vi "PR_CAN_Labview_Demo.vi"() -> ()   [LabVIEW 2017]
uses:
  Fuse25A_Labview/Power-Rider-GUI/CANalystII/PCAN_Driver/ControlCAN.llb/CAN Channel.ctl
  D:/Projects/GUI/Power Rider Wrapper/PowerRiderDLLWrapper.dll
  PowerRiderDLLWrapper.dll
  Fuse25A_Labview/Power-Rider-GUI/CANalystII/PCAN_Driver/ControlCAN.lvlib
panel:
  in  "Channel #":T1 caption="Channel" items=["Channel 1", "Channel 2"]
  in  "Baud":u32(ring)=250000 items=["1M"=1000000, "800K"=800000, "500K"=500000, "250K"=250000, "125K"=125000, "100K"=100000, "83.3K"=83300, "50000"=50000, "20K"=20000, "10K"=10000, "5K"=5000]
  in  "String":string
  out "CommIcon":bool
  in  "Dst add":u16=16
  in  "address":u16=85
  in  "TripType Enum":T2(ring)
  in  "Status Enum":enum16{"OFF", "ON", "ERROR", "FOREVER OFF"}(ring)
  # "Power Rider Demo"
  # "CANalytst-II interface"
  # "ver 1.0"
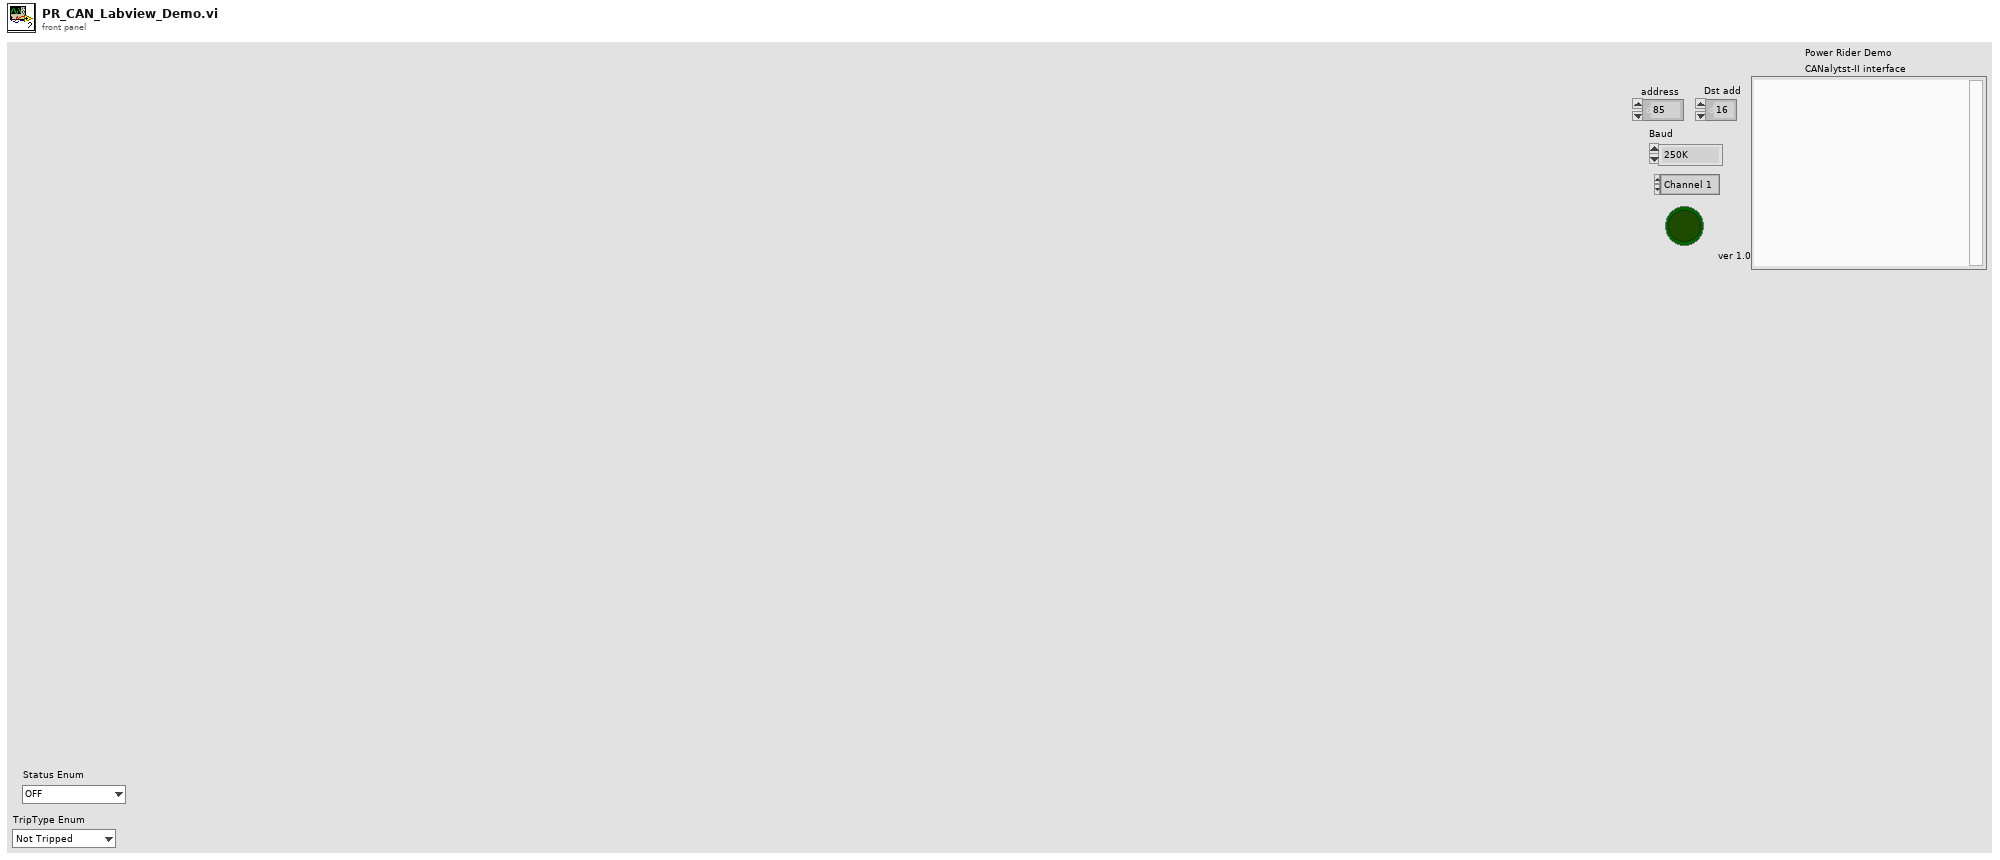
[diagram p1: front panel]
types:
  T1 = typedef "ControlCAN.lvlib/CAN Channel.ctl" = u32
  T2 = enum16{"Not Tripped", "SW Tripped", "Hard Short", "MAX SW Tripped"}
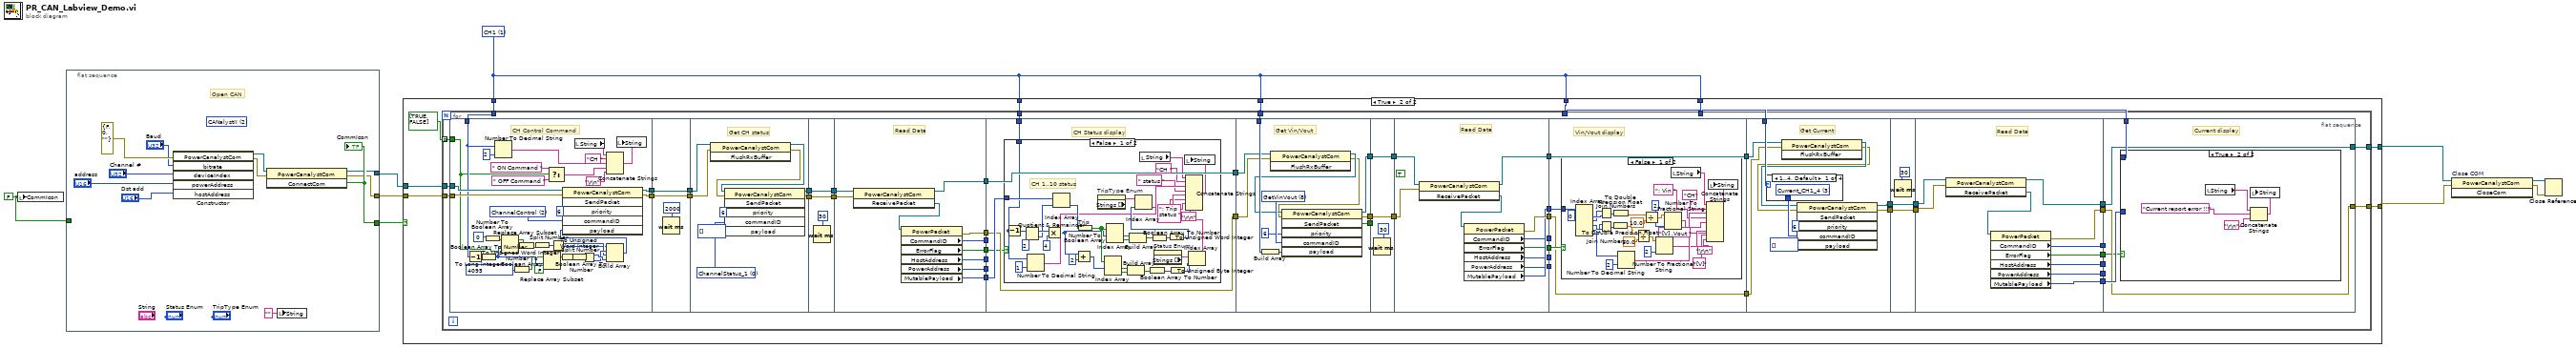
[diagram p0: block diagram]
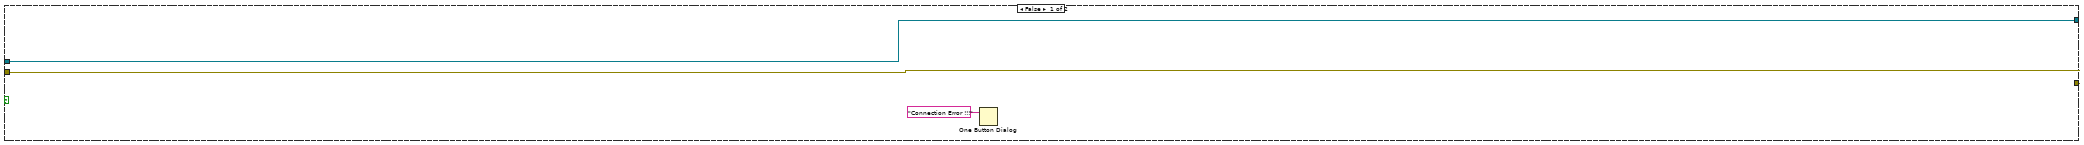
[diagram p2: hidden frame]
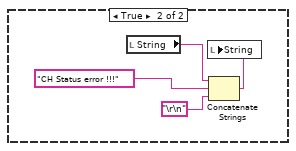
[diagram p3: hidden frame]
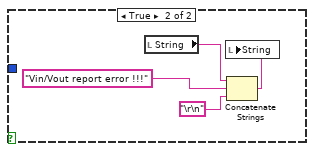
[diagram p4: hidden frame]
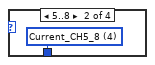
[diagram p5: hidden frame]
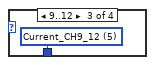
[diagram p6: hidden frame]
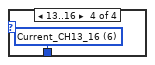
[diagram p7: hidden frame]
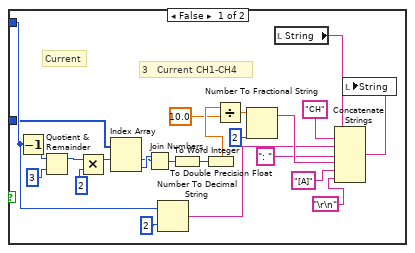
[diagram p8: hidden frame]
diagram:
  w1 = FALSE ("CommIcon")
  w6 = u8 1 items=["CH1"=1, "CH2"=2, "CH3"=3, "CH4"=4, "CH5"=5, "CH6"=6, "CH7"=7, "CH8"=8, "CH9"=9, "CH10"=10, "CH11"=11, "CH12"=12, "CH13"=13, "CH14"=14, "CH15"=15, "CH16"=16] ("Select CH #")
  n1 = local write "CommIcon"(w1) -> ()
  n2 = flat-sequence {
    tunnel: [w12] -> w9
    tunnel: [w11] -> w3
    tunnel: [w10] -> w2
    tunnel: w1 -> [_]
    frame #0 {
      (unwired) u16 2 items=["CANalystII"=2, "TCP Client"=3, "TCP Server"=4, "UDP Client"=5, "Serial COM"=6, "CAN Kvaser"=7] ("COMType 2")
      # "Open CAN"
      n3 = constructor class="PowerCanalystCom"(error in=errorcluster {"status"=FALSE, "code"=0, "source"=""} ("error out"), "bitrate"="Baud", "deviceIndex"="Channel #", "powerAddress"="address", "hostAddress"="Dst add") -> (reference out=w13:refnum<k24>, error out=w14:errorcluster)  [unwired: 2 in, 5 out]
      n4 = invoke class="PowerCanalystCom" method="ConnectCom"(reference=w13, error in=w14) -> (reference out=w10:refnum<k24>, error out=w11:errorcluster, "ConnectCom"=w12:bool)  [unwired: 1 in]
      "CommIcon" <- w12
      n5 = local write "String"("" ("String")) -> ()
    }
  }
  n6 = case shown="True" w9 {
    tunnel: w2 -> [w22 w28]
    tunnel: w3 -> [w23 w27]
    tunnel: w6 -> [_ w33]
    tunnel: w6 -> [_ w32]
    tunnel: w6 -> [_ w31]
    tunnel: w6 -> [_ w30]
    tunnel: w6 -> [_ w29]
    tunnel: [w22 w26] -> w5
    tunnel: [w23 w25] -> w4
    frame False {
      n7 = One Button Dialog(message="Connection Error !!!") -> ()  [unwired: 1 in, 1 out]
    }
    frame True {
      n8 = for {
        tunnel: w33 -> [w34]
        tunnel: w32 -> [w74]
        tunnel: w31 -> [w73]
        tunnel: w30 -> [w72]
        tunnel: w29 -> [w35]
        tunnel: w28 -> [w71]
        tunnel: w27 -> [w70]
        tunnel: [w69] -> w26
        tunnel: [w68] -> w25
        tunnel: bool[] [TRUE, FALSE] -> [w67] mode=indexing
        n9 = flat-sequence {
          tunnel: w70 -> [w99]
          tunnel: [w101] -> w85
          tunnel: [w100] -> w84
          tunnel: w35 -> [w94]
          tunnel: w71 -> [w98]
          tunnel: w67 -> [w90]
          tunnel: w85 -> [w123]
          tunnel: [w123] -> w83
          tunnel: w84 -> [w122]
          tunnel: [w122] -> w82
          tunnel: [w129] -> w66
          tunnel: [w128] -> w64
          tunnel: w83 -> [w127]
          tunnel: w82 -> [w126]
          tunnel: w66 -> [w135]
          tunnel: [w135] -> w65
          tunnel: w64 -> [w134]
          tunnel: [w134] -> w63
          tunnel: w65 -> [w142]
          tunnel: w63 -> [w143]
          tunnel: [w145] -> w81
          tunnel: [w144] -> w80
          tunnel: [w140] -> w79
          tunnel: [w139] -> w48
          tunnel: [w138] -> w47
          tunnel: [w137] -> w46
          tunnel: [w136] -> w45
          tunnel: w81 -> [w148]
          tunnel: w80 -> [w150]
          tunnel: w79 -> [w149]
          tunnel: [w149] -> w78
          tunnel: [w148] -> w77
          tunnel: w34 -> [w147]
          tunnel: w48 -> [w146]
          tunnel: w47 -> [_]
          tunnel: w46 -> [_]
          tunnel: w45 -> [_]
          tunnel: w78 -> [w192]
          tunnel: w77 -> [w190]
          tunnel: w74 -> [w194]
          tunnel: [w196] -> w62
          tunnel: [w195] -> w61
          tunnel: [w193] -> w44
          tunnel: w62 -> [w202]
          tunnel: [w202] -> w59
          tunnel: w61 -> [w201]
          tunnel: [w201] -> w57
          tunnel: w44 -> [_]
          tunnel: [w211] -> w60
          tunnel: w59 -> [w209]
          tunnel: [w208] -> w58
          tunnel: w57 -> [w210]
          tunnel: [w212] -> w56
          tunnel: [w206] -> w43
          tunnel: [w205] -> w42
          tunnel: [w204] -> w41
          tunnel: [w203] -> w40
          tunnel: w60 -> [w216]
          tunnel: [w215] -> w76
          tunnel: w58 -> [w215]
          tunnel: w56 -> [w213]
          tunnel: [w213] -> w75
          tunnel: w43 -> [_]
          tunnel: w42 -> [w214]
          tunnel: w41 -> [_]
          tunnel: w40 -> [_]
          tunnel: w73 -> [w257]
          tunnel: w76 -> [w252]
          tunnel: w75 -> [w251]
          tunnel: [w254] -> w55
          tunnel: [w253] -> w54
          tunnel: w55 -> [w265]
          tunnel: [w265] -> w53
          tunnel: w54 -> [w264]
          tunnel: [w264] -> w51
          tunnel: w53 -> [w273]
          tunnel: [w274] -> w52
          tunnel: w51 -> [w272]
          tunnel: [w270] -> w50
          tunnel: [w275] -> w49
          tunnel: [w269] -> w39
          tunnel: [w268] -> w38
          tunnel: [w267] -> w37
          tunnel: [w266] -> w36
          tunnel: w52 -> [w277]
          tunnel: w50 -> [w278]
          tunnel: w72 -> [w280]
          tunnel: w49 -> [w279]
          tunnel: [w278] -> w69
          tunnel: [w277] -> w68
          tunnel: w39 -> [w276]
          tunnel: w38 -> [_]
          tunnel: w37 -> [_]
          tunnel: w36 -> [_]
          frame #0 {
            w102 = u8 2 items=["ChannelStatus_1"=0, "ChannelControl"=2, "Current_CH1_4"=3, "Current_CH5_8"=4, "Current_CH9_12"=5, "Current_CH13_16"=6, "GetVinVout"=8, "Version_BoardType"=9, "SystemTemp"=10, "SystemParameter"=11, "ChannelParameter"=12, "GetTripEvent"=15, "LogFile"=18, "Configuration"=19, "ProductionData"=20, "BIT"=33, "DiscretePorts"=34, "SerialNumber"=36, "OffsetMeasurement"=37, "PartNumber"=39, "ChannelCombinedStatus_1_CH1_8"=40, "ChannelCombinedStatus_2_CH9_12"=41, "PlotData"=45, "PlotCommand"=46, "InternalData"=47, "KeepAlive"=234, "WakeUp"=250] ("commandID")
            # "CH Control Command"
            n10 = Decrement(x=w94) -> (x-1=w103:u8)
            n11 = To Long Integer(number=w103) -> (32bit integer=w109:i32)
            n12 = Number To Boolean Array(number=u16 0 ("element")) -> (Boolean array=w105:bool[])
            n13 = Number To Decimal String(number=w94, width (-)=i16 2) -> (decimal integer string=w91:string)
            n14 = Replace Array Subset(array=w105, new element=w90, index=w109) -> (w106:bool[])
            n15 = Number To Boolean Array(number=u16 4095 ("mask")) -> (Boolean array=w108:bool[])
            n16 = Boolean Array To Number(Boolean array=w106) -> (number=w107:u32)
            n17 = To Unsigned Word Integer(number=w107) -> (unsigned 16bit integer=w114:u16)
            n18 = Replace Array Subset(array=w108, new element=FALSE ("new element/subarray"), index=w109) -> (w104:bool[])
            n19 = Select(t=" ON Command " ("string"), s=w90, f=" OFF Command " ("string")) -> (s? t:f=w87:string)
            n20 = Split Number(x=w114) -> (hi(x)=w118:u8, lo(x)=w117:u8)
            n21 = Boolean Array To Number(Boolean array=w104) -> (number=w113:u32)
            n22 = To Unsigned Word Integer(number=w113) -> (unsigned 16bit integer=w116:u16)
            n23 = local read "String"() -> (w96:string)
            n24 = Split Number(x=w116) -> (hi(x)=w120:u8, lo(x)=w119:u8)
            n25 = Concatenate Strings(w96, "CH " ("string"), w91, w87, "\r\n") -> (w95:string)
            n26 = Build Array(w117, w119, w118, w120) -> (w115:u8[])
            n27 = invoke class="PowerCanalystCom" method="SendPacket"(reference=w98, error in=w99, "priority"=u8 6, "commandID"=w102, "payload"=w115) -> (reference out=w101:refnum<k24>, error out=w100:errorcluster)  [unwired: 1 in, 4 out]
            n28 = local write "String"(w95) -> ()
          }
          frame #1 {
            n29 = Wait (ms)(milliseconds to wait=u32 2000) -> ()  [unwired: 1 out]
          }
          frame #2 {
            w132 = u8 0 items=["ChannelStatus_1"=0, "ChannelControl"=2, "Current_CH1_4"=3, "Current_CH5_8"=4, "Current_CH9_12"=5, "Current_CH13_16"=6, "GetVinVout"=8, "Version_BoardType"=9, "SystemTemp"=10, "SystemParameter"=11, "ChannelParameter"=12, "GetTripEvent"=15, "LogFile"=18, "Configuration"=19, "ProductionData"=20, "BIT"=33, "DiscretePorts"=34, "SerialNumber"=36, "OffsetMeasurement"=37, "PartNumber"=39, "ChannelCombinedStatus_1_CH1_8"=40, "ChannelCombinedStatus_2_CH9_12"=41, "PlotData"=45, "PlotCommand"=46, "InternalData"=47, "KeepAlive"=234, "WakeUp"=250] ("commandID")
            # "Get CH status"
            n30 = invoke class="PowerCanalystCom" method="FlushRxBuffer"(reference=w127, error in=w126) -> (reference out=w124:refnum<k24>, error out=w125:errorcluster)  [unwired: 1 in, 1 out]
            n31 = invoke class="PowerCanalystCom" method="SendPacket"(reference=w124, error in=w125, "priority"=u8 6, "commandID"=w132, "payload"=u8[] []) -> (reference out=w128:refnum<k24>, error out=w129:errorcluster)  [unwired: 1 in, 4 out]
          }
          frame #3 {
            n32 = Wait (ms)(milliseconds to wait=u32 30) -> ()  [unwired: 1 out]
          }
          frame #4 {
            # "Read Data"
            n33 = invoke class="PowerCanalystCom" method="ReceivePacket"(reference=w143, error in=w142) -> (reference out=w140:refnum<k24>, "ReceivePacket"=w141:refnum<k24>)  [unwired: 1 in, 1 out]
            n34 = property class="PowerPacket"(reference=w141) -> (error out=w145:errorcluster, "CommandID"=w138:u8, "ErrorFlag"=w139:bool, "HostAddress"=w137:u8, "PowerAddress"=w136:u8, "MutablePayload"=w144:u8[])  [unwired: 1 in, 1 out]
          }
          frame #5 {
            # "CH Status display"
            n35 = case shown="False" w146 {
              tunnel: w150 -> [w157 _]
              tunnel: w147 -> [w154 _]
              frame False {
                # "CH 1..10 status"
                n36 = Decrement(x=w154) -> (x-1=w151:u8)
                n37 = Quotient & Remainder(x=w151, y=2) -> (x-y*floor(x/y)=w167:i32, floor(x/y)=w166:i32)
                n38 = Number To Decimal String(number=w154, width (-)=i16 1) -> (decimal integer string=w170:string)
                n39 = Multiply(x=w167, y=u8 4) -> (x*y=w165:i32)
                n40 = Index Array(array=w157, index=w166) -> (element=w172:u8)
                n41 = Add(x=w165, y=u8 2) -> (x+y=w164:i32)
                n42 = Number To Boolean Array "Trip"(number=w172) -> (Boolean array=w171:bool[])
                n43 = property on="TripType Enum" class="Enum (strict)"() -> ("Strings []"=w181:string[])  [unwired: 2 in, 2 out]
                n44 = Index Array(array=w171, index #1=w164) -> (element #1=w180:bool, element #2=w179:bool)  [unwired: 1 in]
                n45 = Index Array(array=w171, index #1=w165) -> (element #1=w177:bool, element #2=w178:bool)  [unwired: 1 in]
                n46 = Build Array(w180, w179) -> (w176:bool[])
                n47 = Build Array(w177, w178) -> (w175:bool[])
                n48 = local read "String"() -> (w153:string)
                n49 = Boolean Array To Number(Boolean array=w176) -> (number=w174:u32)
                n50 = Boolean Array To Number(Boolean array=w175) -> (number=w173:u32)
                n51 = property on="Status Enum" class="Enum (strict)"() -> ("Strings []"=w182:string[])  [unwired: 2 in, 2 out]
                n52 = To Unsigned Word Integer(number=w173) -> (unsigned 16bit integer=w183:u16)
                n53 = Index Array(array=w181, index=w183) -> (element=w169:string)
                n54 = To Unsigned Byte Integer(number=w174) -> (unsigned 8bit integer=w184:u8)
                n55 = Index Array(array=w182, index=w184) -> (element=w168:string)
                n56 = Concatenate Strings(w153, "CH " ("string"), w170, " status ", w168, "; Trip status ", w169, "\r\n") -> (w156:string)
                n57 = local write "String"(w156) -> ()
              }
              frame True {
                n58 = local read "String"() -> (w187:string)
                n59 = Concatenate Strings(w187, "CH Status error !!!" ("string"), "\r\n") -> (w188:string)
                n60 = local write "String"(w188) -> ()
              }
            }
          }
          frame #6 {
            w198 = u8 8 items=["ChannelStatus_1"=0, "ChannelControl"=2, "Current_CH1_4"=3, "Current_CH5_8"=4, "Current_CH9_12"=5, "Current_CH13_16"=6, "GetVinVout"=8, "Version_BoardType"=9, "SystemTemp"=10, "SystemParameter"=11, "ChannelParameter"=12, "GetTripEvent"=15, "LogFile"=18, "Configuration"=19, "ProductionData"=20, "BIT"=33, "DiscretePorts"=34, "SerialNumber"=36, "OffsetMeasurement"=37, "PartNumber"=39, "ChannelCombinedStatus_1_CH1_8"=40, "ChannelCombinedStatus_2_CH9_12"=41, "PlotData"=45, "PlotCommand"=46, "InternalData"=47, "KeepAlive"=234, "WakeUp"=250] ("commandID")
            # "Get Vin/Vout"
            n61 = Build Array(w194) -> (w199:u8[])
            n62 = invoke class="PowerCanalystCom" method="FlushRxBuffer"(reference=w192, error in=w190) -> (reference out=w191:refnum<k24>, error out=w189:errorcluster)  [unwired: 1 in, 1 out]
            n63 = invoke class="PowerCanalystCom" method="SendPacket"(reference=w191, error in=w189, "priority"=u8 6, "commandID"=w198, "payload"=w199) -> (reference out=w196:refnum<k24>, error out=w195:errorcluster, "SendPacket"=w193:bool)  [unwired: 1 in, 3 out]
          }
          frame #7 {
            n64 = Wait (ms)(milliseconds to wait=u32 30) -> ()  [unwired: 1 out]
          }
          frame #8 {
            (unwired) TRUE
            # "Read Data"
            n65 = invoke class="PowerCanalystCom" method="ReceivePacket"(reference=w209, error in=w210) -> (reference out=w208:refnum<k24>, "ReceivePacket"=w207:refnum<k24>)  [unwired: 1 in, 1 out]
            n66 = property class="PowerPacket"(reference=w207) -> (error out=w212:errorcluster, "CommandID"=w206:u8, "ErrorFlag"=w205:bool, "HostAddress"=w204:u8, "PowerAddress"=w203:u8, "MutablePayload"=w211:u8[])  [unwired: 1 in, 1 out]
          }
          frame #9 {
            # "Vin/Vout display"
            n67 = case shown="False" w214 {
              tunnel: w216 -> [w220 _]
              frame False {
                n68 = Index Array(array=w220, index #1=0 ("index")) -> (element #1=w242:u8, element #2=w241:u8, element #3=w240:u8, element #4=w239:u8, element #5=w236:u8)  [unwired: 4 in]
                n69 = Join Numbers(hi=w241, lo=w242) -> ((hi.lo)=w243:u16)
                n70 = Join Numbers(hi=w239, lo=w240) -> ((hi.lo)=w244:u16)
                n71 = To Double Precision Float(number=w244) -> (double precision float=w237:dbl)
                n72 = To Double Precision Float(number=w243) -> (double precision float=w238:dbl)
                n73 = Number To Decimal String(number=w236, width (-)=i16 2) -> (decimal integer string=w235:string)
                n74 = Divide(x=w237, y=10.0) -> (x/y=w232:dbl)
                n75 = Divide(x=w238, y=10.0) -> (x/y=w234:dbl)
                n76 = Number To Fractional String(number=w232, precision (6)=i16 2) -> (F-format string=w231:string)  [unwired: 2 in]
                n77 = Number To Fractional String(number=w234, precision (6)=i16 2) -> (F-format string=w233:string)  [unwired: 2 in]
                n78 = local read "String"() -> (w218:string)
                n79 = Concatenate Strings(w218, "CH" ("string"), w235, ": Vin " ("string"), w233, "[V] ,Vout " ("string"), w231, "[V]" ("string"), "\r\n") -> (w219:string)
                n80 = local write "String"(w219) -> ()
              }
              frame True {
                n81 = local read "String"() -> (w247:string)
                n82 = Concatenate Strings(w247, "Vin/Vout report error !!!" ("string"), "\r\n") -> (w248:string)
                n83 = local write "String"(w248) -> ()
              }
            }
          }
          frame #10 {
            # "Get Current"
            n84 = case shown="1..4, Default" w257 {
              tunnel: [w259 w260 w261 w262] -> w258
              frame 1..4, Default {
                w259 = u8 3 items=["ChannelStatus_1"=0, "ChannelControl"=2, "Current_CH1_4"=3, "Current_CH5_8"=4, "Current_CH9_12"=5, "Current_CH13_16"=6, "GetVinVout"=8, "Version_BoardType"=9, "SystemTemp"=10, "SystemParameter"=11, "ChannelParameter"=12, "GetTripEvent"=15, "LogFile"=18, "Configuration"=19, "ProductionData"=20, "BIT"=33, "DiscretePorts"=34, "SerialNumber"=36, "OffsetMeasurement"=37, "PartNumber"=39, "ChannelCombinedStatus_1_CH1_8"=40, "ChannelCombinedStatus_2_CH9_12"=41, "PlotData"=45, "PlotCommand"=46, "InternalData"=47, "KeepAlive"=234, "WakeUp"=250] ("commandID")
              }
              frame 5..8 {
                w260 = u8 4 items=["ChannelStatus_1"=0, "ChannelControl"=2, "Current_CH1_4"=3, "Current_CH5_8"=4, "Current_CH9_12"=5, "Current_CH13_16"=6, "GetVinVout"=8, "Version_BoardType"=9, "SystemTemp"=10, "SystemParameter"=11, "ChannelParameter"=12, "GetTripEvent"=15, "LogFile"=18, "Configuration"=19, "ProductionData"=20, "BIT"=33, "DiscretePorts"=34, "SerialNumber"=36, "OffsetMeasurement"=37, "PartNumber"=39, "ChannelCombinedStatus_1_CH1_8"=40, "ChannelCombinedStatus_2_CH9_12"=41, "PlotData"=45, "PlotCommand"=46, "InternalData"=47, "KeepAlive"=234, "WakeUp"=250] ("commandID")
              }
              frame 9..12 {
                w261 = u8 5 items=["ChannelStatus_1"=0, "ChannelControl"=2, "Current_CH1_4"=3, "Current_CH5_8"=4, "Current_CH9_12"=5, "Current_CH13_16"=6, "GetVinVout"=8, "Version_BoardType"=9, "SystemTemp"=10, "SystemParameter"=11, "ChannelParameter"=12, "GetTripEvent"=15, "LogFile"=18, "Configuration"=19, "ProductionData"=20, "BIT"=33, "DiscretePorts"=34, "SerialNumber"=36, "OffsetMeasurement"=37, "PartNumber"=39, "ChannelCombinedStatus_1_CH1_8"=40, "ChannelCombinedStatus_2_CH9_12"=41, "PlotData"=45, "PlotCommand"=46, "InternalData"=47, "KeepAlive"=234, "WakeUp"=250] ("commandID")
              }
              frame 13..16 {
                w262 = u8 6 items=["ChannelStatus_1"=0, "ChannelControl"=2, "Current_CH1_4"=3, "Current_CH5_8"=4, "Current_CH9_12"=5, "Current_CH13_16"=6, "GetVinVout"=8, "Version_BoardType"=9, "SystemTemp"=10, "SystemParameter"=11, "ChannelParameter"=12, "GetTripEvent"=15, "LogFile"=18, "Configuration"=19, "ProductionData"=20, "BIT"=33, "DiscretePorts"=34, "SerialNumber"=36, "OffsetMeasurement"=37, "PartNumber"=39, "ChannelCombinedStatus_1_CH1_8"=40, "ChannelCombinedStatus_2_CH9_12"=41, "PlotData"=45, "PlotCommand"=46, "InternalData"=47, "KeepAlive"=234, "WakeUp"=250] ("commandID")
              }
            }
            n85 = invoke class="PowerCanalystCom" method="FlushRxBuffer"(reference=w252, error in=w251) -> (reference out=w250:refnum<k24>, error out=w249:errorcluster)  [unwired: 1 in, 1 out]
            n86 = invoke class="PowerCanalystCom" method="SendPacket"(reference=w250, error in=w249, "priority"=u8 6, "commandID"=w258, "payload"=u8[] []) -> (reference out=w253:refnum<k24>, error out=w254:errorcluster)  [unwired: 1 in, 4 out]
          }
          frame #11 {
            n87 = Wait (ms)(milliseconds to wait=u32 30) -> ()  [unwired: 1 out]
          }
          frame #12 {
            # "Read Data"
            n88 = invoke class="PowerCanalystCom" method="ReceivePacket"(reference=w272, error in=w273) -> (reference out=w270:refnum<k24>, "ReceivePacket"=w271:refnum<k24>)  [unwired: 1 in, 1 out]
            n89 = property class="PowerPacket"(reference=w271) -> (error out=w274:errorcluster, "CommandID"=w266:u8, "ErrorFlag"=w269:bool, "HostAddress"=w268:u8, "PowerAddress"=w267:u8, "MutablePayload"=w275:u8[])  [unwired: 1 in, 1 out]
          }
          frame #13 {
            # "Current display"
            n90 = case shown="True" w276 {
              tunnel: w280 -> [w285 _]
              tunnel: w279 -> [w284 _]
              frame False {
                # "3   Current CH1-CH4"
                # "Current"
                n91 = Decrement(x=w285) -> (x-1=w286:u8)
                n92 = Quotient & Remainder(x=w286, y=u8 3) -> (x-y*floor(x/y)=w300:u8)  [unwired: 1 out]
                n93 = Multiply(x=w300, y=u8 2) -> (x*y=w299:u8)
                n94 = Index Array(array=w284, index #1=w299) -> (element #1=w297:u8, element #2=w298:u8)  [unwired: 1 in]
                n95 = Join Numbers(hi=w298, lo=w297) -> ((hi.lo)=w301:u16)
                n96 = Number To Decimal String(number=w285, width (-)=i16 2) -> (decimal integer string=w295:string)
                n97 = To Word Integer(number=w301) -> (16bit integer=w303:i16)
                n98 = To Double Precision Float(number=w303) -> (double precision float=w302:dbl)
                n99 = Divide(x=w302, y=10.0) -> (x/y=w296:dbl)
                n100 = Number To Fractional String(number=w296, precision (6)=i16 2) -> (F-format string=w304:string)  [unwired: 2 in]
                n101 = local read "String"() -> (w281:string)
                n102 = Concatenate Strings(w281, "CH" ("string"), w295, ": " ("string"), w304, "[A]" ("string"), "\r\n") -> (w283:string)
                n103 = local write "String"(w283) -> ()
              }
              frame True {
                n104 = local read "String"() -> (w307:string)
                n105 = Concatenate Strings(w307, "Current report error !!!" ("string"), "\r\n") -> (w308:string)
                n106 = local write "String"(w308) -> ()
              }
            }
          }
        }
      }
    }
  }
  n107 = invoke on="Close COM" class="PowerCanalystCom" method="CloseCom"(reference=w5, error in=w4) -> (reference out=w8:refnum<k24>, error out=w7:errorcluster)  [unwired: 1 in, 1 out]
  n108 = Close Reference(reference=w8, error in (no error)=w7) -> ()  [unwired: 1 out]
